vi "Create Global MetaData Channel - Array - Type Cast.vi"(8 "error in (no error)":errorcluster, 9 "settings":T2, 10 "channel name":string, 11 "instrument addon refnum in":T1=18446744073709551615 format="%.0x") -> (0 "error out":errorcluster, 1 "channel refnums":T1[](array[typedef]) format="%.0x", 2 "array refnum":T1=18446744073709551615 format="%.0x", 3 "instrument addon refnum out":T1=18446744073709551615 format="%.0x")   [LabVIEW 2019, in "Instrument Addon Scripting API.lvlib"]
doc: "Creates new channels in the Global MetaData Channels section of the specified Instrument Addon Custom Device."
uses:
  Instrument Addon Scripting API.lvlib
  <vilib>/NI VeriStand/Custom Device API/Custom Device Item Ref.ctl
  TypeDefs/Array Type Cast Settings.ctl
  TypeDefs/Array Element.ctl
  Addon/Addon Shared/Types/Type Cast Type.ctl
  Addon/Addon Shared/Types/Endian.ctl
  Addon/Addon Shared/Types/MetaData Parameters.ctl
  Addon/Addon Shared/Types/Protocol Data Type.ctl
  Addon/Addon Shared/Types/Metadata Channel Type.ctl
  Addon/Addon Shared/SubVIs/Constants.vi
  Addon/Addon Shared/Instrument Addon Shared.lvlib
  <vilib>/NI VeriStand/Custom Device API/Custom Device API.lvlib
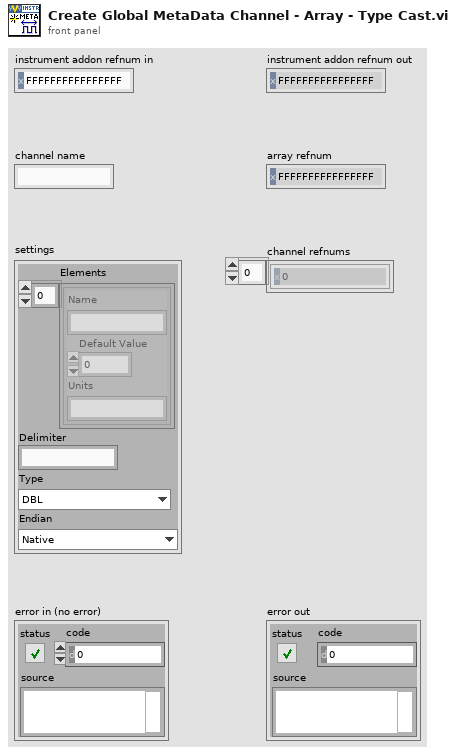
[diagram p1: front panel]
types:
  T1 = typedef "Custom Device API.lvlib/Custom Device Item Ref.ctl" = u64
  T2 = typedef "Instrument Addon Scripting API.lvlib/Array Type Cast Settings.ctl" = cluster{"Elements":T3[], "Delimiter":string, "Type":T4, "Endian":T5}
  T3 = typedef "Instrument Addon Scripting API.lvlib/Array Element.ctl" = cluster{"Name":string, "Default Value":dbl, "Units":string}
  T4 = typedef "Instrument Addon Shared.lvlib/Type Cast Type.ctl" = enum16{"DBL", "SGL", "U64", "U32", "U16", "U8", "I64", "I32", "I16", "I8"}
  T5 = typedef "Instrument Addon Shared.lvlib/Endian.ctl" = enum16{"Native", "Little", "Big"}
  T6 = typedef "Instrument Addon Shared.lvlib/Metadata Channel Type.ctl" = enum16{"Enumerated List", "Format", "Type Cast"}
  T7 = typedef "Instrument Addon Shared.lvlib/Protocol Data Type.ctl" = enum16{"Single Channel", "Array"}
  T8 = typedef "Instrument Addon Shared.lvlib/MetaData Parameters.ctl" = cluster{"Data Type":T7, "Channel Type":T6, "List":string[], "Format String":string, "Type":T4, "Delimiter":string, "Endian":T5}
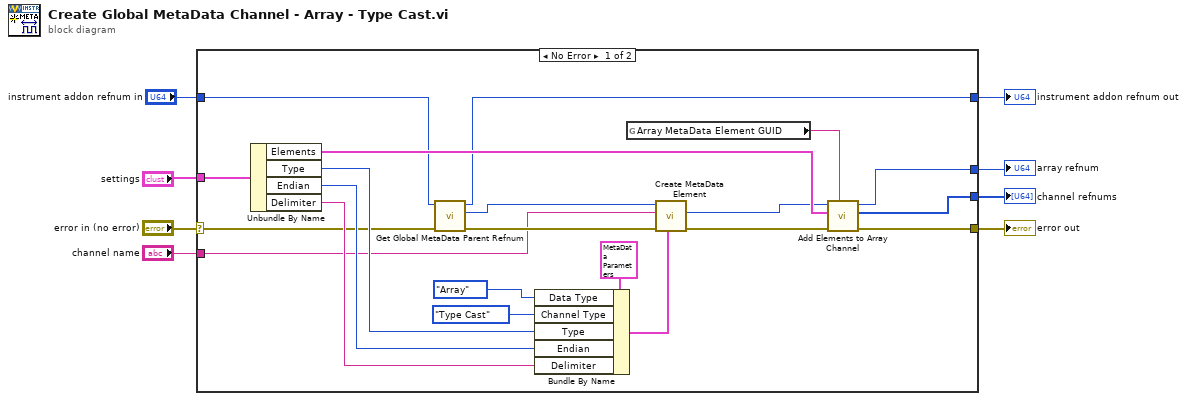
[diagram p0: block diagram]
diagram:
  n1 = case shown="No Error" "error in (no error)" {
    selector: "error in (no error)" -> [w14 w30]
    tunnel: "instrument addon refnum in" -> [w13 w31]
    tunnel: [w12 w31] -> w7
    tunnel: "channel name" -> [w10 _]
    tunnel: "settings" -> [w25 _]
    tunnel: [w23 w30] -> w5
    tunnel: [w17 _] -> w2
    tunnel: [w16 _] -> w1
    frame No Error {
      n2 = Unbundle By Name(w25) -> ("Elements"=w19:T3[], "Type"=w22:T4, "Endian"=w21:T5, "Delimiter"=w20:string)
      n3 = call "Get Global MetaData Parent Refnum.vi"("error in (no error)"=w14, "instrument addon refnum in"=w13) -> ("error out"=w15:errorcluster, "global metadata section refnum"=w11:T1, "instrument addon refnum out"=w12:T1)  [unwired: 7 in]
      n4 = Bundle By Name(cluster=T8 {"Data Type"=enum."Single Channel", "Channel Type"=enum."Format", "List"=[], "Format String"="%.3g", "Type"=enum."SGL", "Delimiter"="", "Endian"=enum."Native"} ("MetaData Parameters"), "Data Type"=Protocol_Data_Type."Array", "Channel Type"=Metadata_Channel_Type."Type Cast", "Type"=w22, "Endian"=w21, "Delimiter"=w20) -> (w26:T8)
      n5 = global read "Constants.vi" "Array MetaData Element GUID"() -> (w9:string)
      n6 = call "Create MetaData Element.vi"("MetaData Parameters"=w26, "error in (no error)"=w15, "Name"=w10, "Refnum In"=w11) -> ("error out"=w24:errorcluster, "Channel Refnum"=w18:T1)  [unwired: 5 in, 1 out]
      n7 = call "Add Elements to Array Channel.vi"("array element GUID"=w9, "error in (no error)"=w24, "array elements"=w19, "array refnum in"=w18) -> ("error out"=w23:errorcluster, "channel refnums"=w17:T1[], "array refnum out"=w16:T1)  [unwired: 5 in]
    }
    frame Error {
    }
  }
  "instrument addon refnum out" <- w7
  "error out" <- w5
  "channel refnums" <- w2
  "array refnum" <- w1
